vi "Tools整体图.vi"() -> ()   [LabVIEW 2014]
panel:
  in  "Cut":bool
  in  "Copy":bool
  in  "Configure":bool
  in  "Compile":bool
  in  "Clipboard":bool
  in  "Clear history":bool
  in  "Bug":bool
  in  "Attach":bool
  in  "Alarm":bool
  in  "Write":bool
  in  "Words":bool
  in  "Wizard":bool
  in  "Utilities":bool
  in  "Trash":bool
  in  "System":bool
  in  "Shred":bool
  in  "Services":bool
  in  "Semaphore":bool
  in  "Safe":bool
  in  "Run":bool
  in  "Quiz":bool
  in  "Quick print":bool
  in  "Print":bool
  in  "Print frame":bool
  in  "Paste":bool
  in  "Package system":bool
  in  "Organizer":bool
  in  "Notes":bool
  in  "Notepad":bool
  in  "Misc":bool
  in  "Lock":bool
  in  "Kate":bool
  in  "Info":bool
  in  "History":bool
  in  "Help":bool
  in  "Help index":bool
  in  "Help center":bool
  in  "Editor":bool
  in  "Edit":bool
  in  "Edit config":bool
  in  "Dock":bool
  in  "Disable alarm":bool
  in  "Dictionary":bool
  in  "Develop":bool
  in  "Delete":bool
  in  "Date":bool
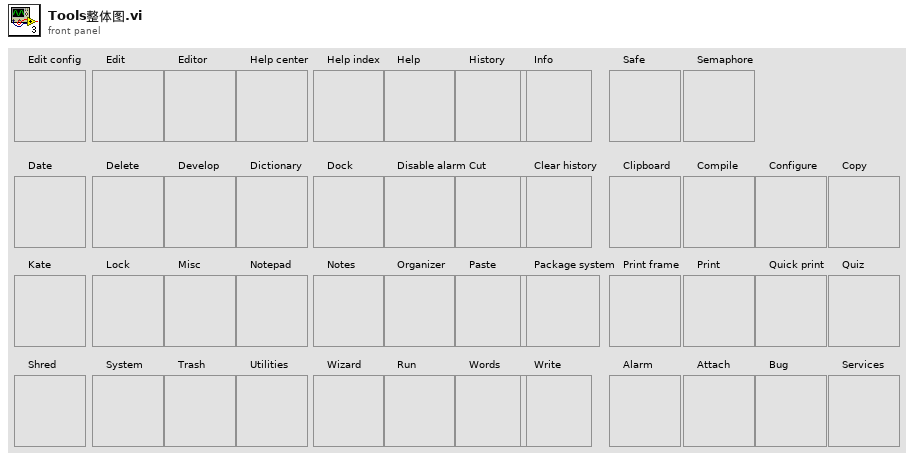
[diagram p1: front panel]
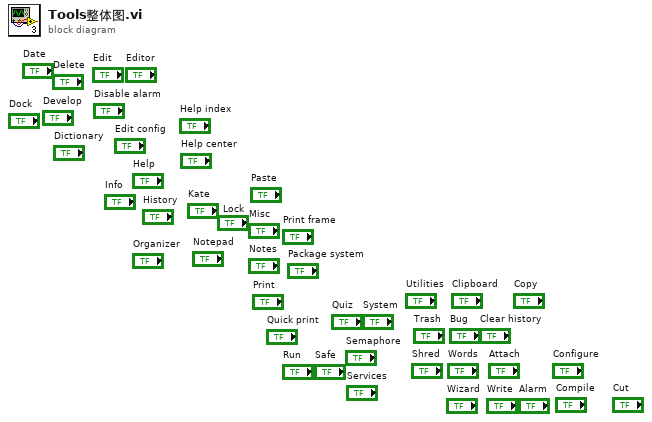
[diagram p0: block diagram]
diagram:
